vi "Finalize Turn.vi"(7 "Move State":T1={"InPlayPos Dict"=variant(i32[] [])}, 8 "error in (no error)":errorcluster, 10 "Turn Penalty[team]":i32[](array[numeric]), 11 "Maze 2.0 in":refnum<class "Maze 2.0.lvclass">) -> (0 "error out":errorcluster, 3 "Maze 2.0 out":refnum<class "Maze 2.0.lvclass">)   [LabVIEW 2014, in "Maze 2.0.lvclass"]
uses:
  Maze 2.0.lvclass
  Move State Cluster.ctl
  Maze 2.0.lvclass/Maze 2.0.ctl
  InPlay Position Cluster.ctl
  Runner/Runner.lvclass
  Runner Cluster.ctl
panel:
  # "What information:\n\nfor in play squares:\nID of players in square\nIs attacked."
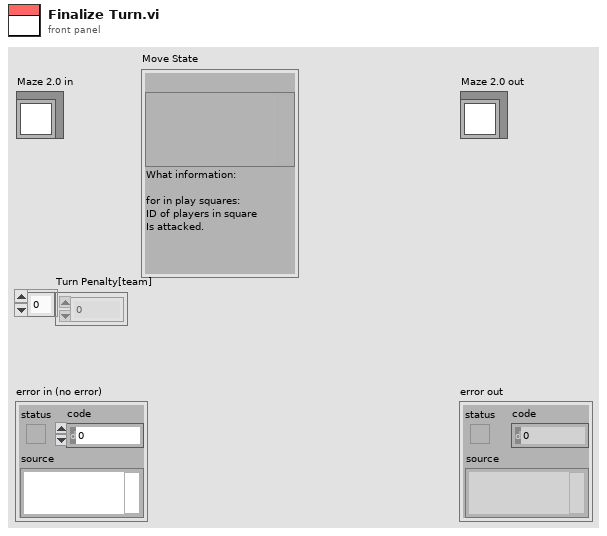
[diagram p1: front panel]
types:
  T1 = typedef "Maze 2.0.lvclass/Move State Cluster.ctl" = cluster{"InPlayPos Dict":variant}
  T2 = typedef "Maze 2.0.lvclass/InPlay Position Cluster.ctl" = cluster{"Attacked?":bool, "player[i]":cluster{"TeamIdx":i32, "NextMove":i32, "RunnerRef":refnum<data-value>, "Player #":i32}[]}
  T3 = typedef "Maze 2.0.lvclass/Runner Cluster.ctl" = cluster{"Alive?":bool, "RunnerRef":refnum<data-value>, "TeamIdx":i32, "Player #":i32, "NextPlay":u32}
  T4 = cluster{"TeamIdx":i32, "NextMove":i32, "RunnerRef":refnum<data-value>, "Player #":i32}[]
  T5 = cluster{"TeamIdx":i32, "NextMove":i32, "RunnerRef":refnum<data-value>, "Player #":i32}
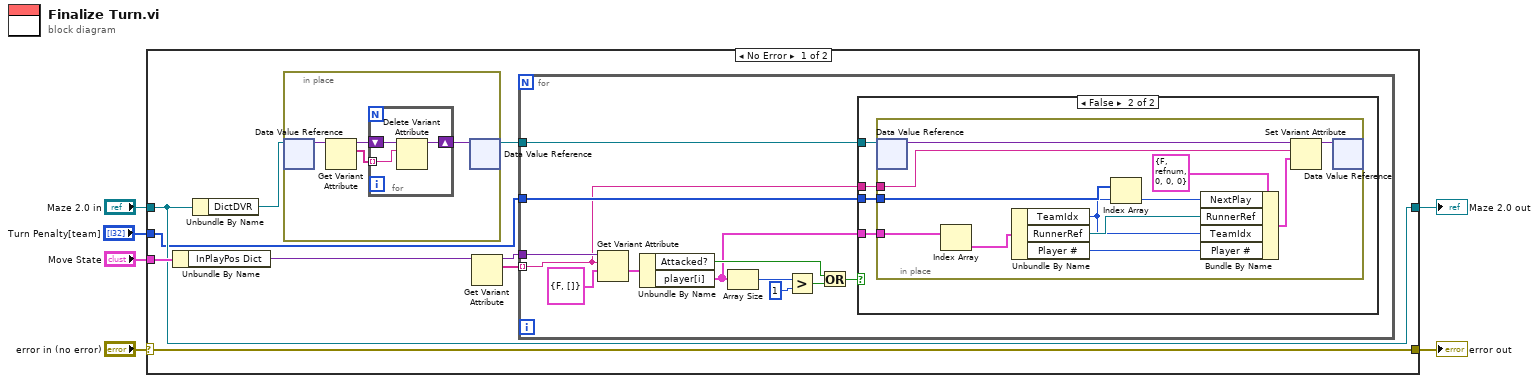
[diagram p0: block diagram]
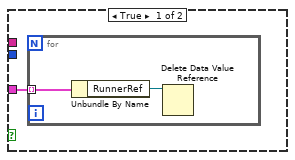
[diagram p2: hidden frame]
diagram:
  n1 = case shown="No Error" "error in (no error)" {
    selector: "error in (no error)" -> [w15 w55]
    tunnel: [w15 w55] -> w5
    tunnel: [w10 w54] -> w3
    tunnel: "Maze 2.0 in" -> [w10 w54]
    tunnel: "Move State" -> [w14 _]
    tunnel: "Turn Penalty[team]" -> [w9 _]
    frame No Error {
      n2 = Unbundle By Name(w14) -> ("InPlayPos Dict"=w13:variant)
      n3 = Unbundle By Name(w10) -> ("DictDVR"=w8:refnum<data-value>)
      n4 = in-place {
        n5 = in-place-dvr #1(w8) -> (w18:variant)  [unwired: 1 out]
        n6 = Get Variant Attribute(Variant=w18) -> (duplicate Variant=w17:variant, names=w16:string[])  [unwired: 3 in, 2 out]
        n7 = for {
          shift-right: [w22] -> w19
          shift-left: w17 -> [w21]
          tunnel: w16 -> [w20] mode=indexing
          n8 = Delete Variant Attribute(6:w20, 7:w21) -> (3:w22:variant)  [unwired: 1 in, 2 out]
        }
        n9 = in-place-dvr #1(w19) -> (w7:refnum<data-value>)  [unwired: 1 out]
      }
      n10 = Get Variant Attribute(Variant=w13) -> (duplicate Variant=w11:variant, names=w12:string[])  [unwired: 3 in, 2 out]
      n11 = for {
        tunnel: w12 -> [w23] mode=indexing
        tunnel: w11 -> [w34]
        tunnel: w7 -> [w33]
        tunnel: w9 -> [w29]
        n12 = Get Variant Attribute(Variant=w34, name=w23, default value (empty Variant)=T2 {"Attacked?"=FALSE, "player[i]"=[]} ("InPlay Position Cluster")) -> (value=w32:T2)  [unwired: 1 in, 3 out]
        n13 = Unbundle By Name(w32) -> ("Attacked?"=w30:bool, "player[i]"=w28:T4)
        n14 = Array Size(array=w28) -> (size(s)=w27:i32)
        n15 = Greater?(x=w27, y=1) -> (0:w24:bool)
        n16 = Or(x=w30, y=w24) -> (x .or. y?=w25:bool)
        n17 = case shown="False" w25 {
          tunnel: w33 -> [_ w41]
          tunnel: w28 -> [w35 w40]
          tunnel: w29 -> [_ w39]
          tunnel: w23 -> [_ w38]
          frame True {
            n18 = for {
              tunnel: w35 -> [w37] mode=indexing
              n19 = Unbundle By Name(w37) -> ("RunnerRef"=w36:refnum<data-value>)
              n20 = Delete Data Value Reference(data value reference=w36) -> ()  [unwired: 1 in, 2 out]
            }
          }
          frame False {
            n21 = in-place {
              in-place-border: w40 -> [w51]
              in-place-border: w39 -> [w50]
              in-place-border: w38 -> [w42]
              n22 = in-place-dvr #2(w41) -> (w53:variant)  [unwired: 1 out]
              n23 = Index Array(array=w51) -> (element=w44:T5)  [unwired: 1 in]
              n24 = Unbundle By Name(w44) -> ("TeamIdx"=w45:i32, "RunnerRef"=w46:refnum<data-value>, "Player #"=w43:i32)
              n25 = Index Array(array=w50, index=w45) -> (element=w49:i32)
              n26 = Bundle By Name(cluster=T3 {"Alive?"=FALSE, "RunnerRef"=refnum, "TeamIdx"=0, "Player #"=0, "NextPlay"=0} ("Cluster"), "NextPlay"=w49, "RunnerRef"=w46, "TeamIdx"=w45, "Player #"=w43) -> (w48:T3)
              n27 = Set Variant Attribute(Variant=w53, name=w42, value=w48) -> (Variant out=w52:variant)  [unwired: 1 in, 2 out]
              n28 = in-place-dvr #2(w52) -> ()  [unwired: 2 out]
            }
          }
        }
      }
    }
    frame Error {
    }
  }
  "error out" <- w5
  "Maze 2.0 out" <- w3
